vi "Search Object List.vi"(10 "object ID":u8 format="%x", 11 "objects":cluster{"object ID":u8, "value":string}[](array[cluster]) {"object ID" format="%x"}) -> (2 "object":cluster{"object ID":u8, "value":string} {"object ID" format="%x"}, 3 "found?":bool, 5 "index":i32)   [LabVIEW 2020, in "SubVIs.lvlib" / "Device Data Model.lvclass"]
doc: "This VI looks for a specific object in the full list."
uses:
  <vilib>/Modbus/subvis/Data and Functions/Device Data Model/Device Data Model.lvclass
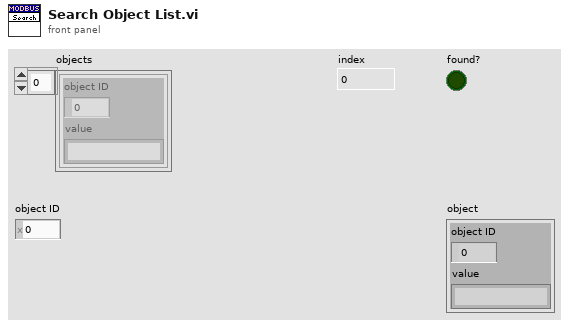
[diagram p1: front panel]
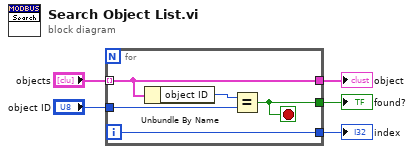
[diagram p0: block diagram]
diagram:
  n1 = for {
    tunnel: "objects" -> [w8] mode=indexing
    tunnel: "object ID" -> [w9]
    tunnel: [w8] -> w3
    tunnel: [w7] -> w2
    tunnel: [w6] -> w1
    i -> [w6]
    stop <- w7 stop-if-true
    n2 = Unbundle By Name(w8) -> ("object ID"=w10:u8)
    n3 = Equal?(x=w10, y=w9) -> (x = y?=w7:bool)
  }
  "found?" <- w2
  "object" <- w3
  "index" <- w1
